vi "save_xml.vi"(8 "error in":errorcluster, 10 "base path":path, 11 "Camera Setup":T1={"Analog Gain (0-5)"=4, "Exposure Time"=0.01, "EM Gain (0-255)"=0, "Trigger Polarity"="ATP P", "External Trigger Mode"="ATP P", "Scan Speed"="EMD E", "External Trigger Source"="SSP H", "Scan Mode"="ESC B", "Super Pixel Binning\n(if enabled in Scan Mode)"="SMD N", "Camera Sub-array acquisition region\n(if enabled in scan mode)"={"Left"=0, "Top"=0, "Width"=0, "Height"=0}, "Use camera?"=FALSE, "# image buffers"=100, "shots per measurement"=100, "Force images to U16"=FALSE, "Low Light Sensitivity"="LLS 0", "cooling"="CSW F", "fan"="FAN F", "Frame Grabber acquisition region"={"Left"=0, "Top"=0, "Right"=0, "Bottom"=0}} {"Frame Grabber acquisition region"."Bottom" max=512 step=1; "Frame Grabber acquisition region"."Right" max=512 step=1; "Frame Grabber acquisition region"."Top" max=512 step=1; "Frame Grabber acquisition region"."Left" max=512 step=1; "shots per measurement" min=0 step=1; "# image buffers" min=0 step=1; "Camera Sub-array acquisition region\n(if enabled in scan mode)"."Height" min=16 max=512 step=16; "Camera Sub-array acquisition region\n(if enabled in scan mode)"."Width" min=16 max=512 step=16; "Camera Sub-array acquisition region\n(if enabled in scan mode)"."Top" max=496 step=16; "Camera Sub-array acquisition region\n(if enabled in scan mode)"."Left" max=496 step=16; "Analog Gain (0-5)" max=5 step=1}) -> (0 "error out":errorcluster)   [LabVIEW 2013, in "Hamamatsu_C9100-13.lvclass"]
uses:
  Hamamatsu_C9100-13.lvclass
  <vilib>/Utility/xml.llb/Write to XML File(string).vi
  camera_setup.ctl
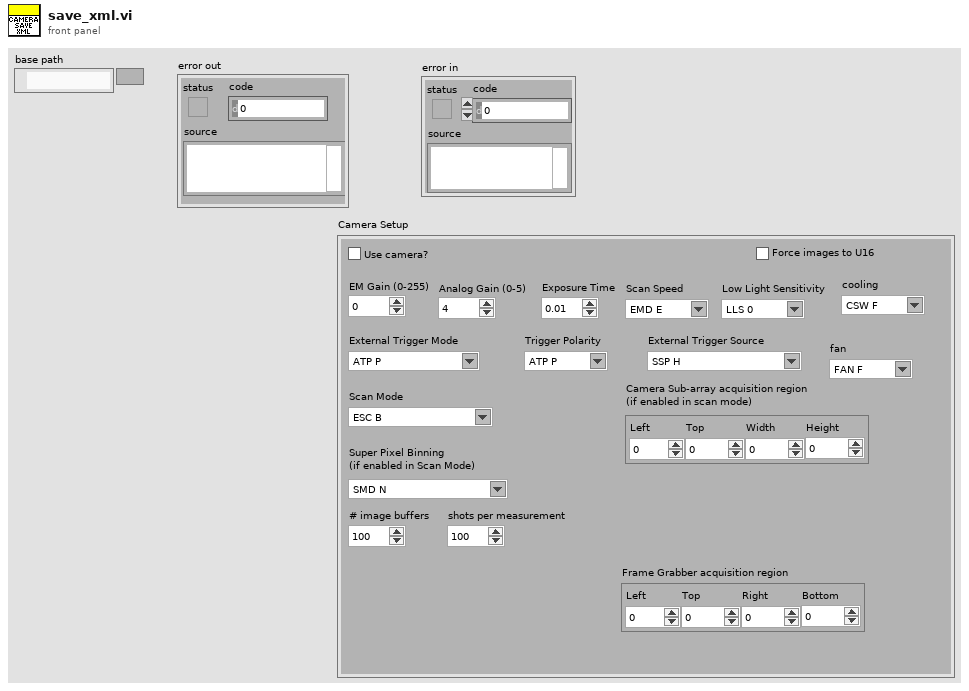
[diagram p1: front panel]
types:
  T1 = typedef "Hamamatsu_C9100-13.lvclass/camera_setup.ctl" = cluster{"Analog Gain (0-5)":u8, "Exposure Time":dbl, "EM Gain (0-255)":u8, "Trigger Polarity":string, "External Trigger Mode":string, "Scan Speed":string, "External Trigger Source":string, "Scan Mode":string, "Super Pixel Binning\n(if enabled in Scan Mode)":string, "Camera Sub-array acquisition region\n(if enabled in scan mode)":cluster{"Left":u16, "Top":u16, "Width":u16, "Height":u16}, "Use camera?":bool, "# image buffers":i32, "shots per measurement":i32, "Force images to U16":bool, "Low Light Sensitivity":string, "cooling":string, "fan":string, "Frame Grabber acquisition region":cluster{"Left":i32, "Top":i32, "Right":i32, "Bottom":i32}}
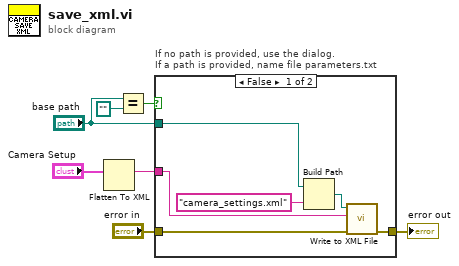
[diagram p0: block diagram]
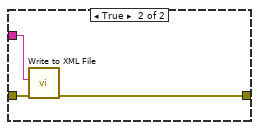
[diagram p2: hidden frame]
diagram:
  n1 = Flatten To XML(anything="Camera Setup") -> (xml string=w2:string)
  n2 = Equal?(x="base path", y=path "") -> (x = y?=w5:bool)
  n3 = case "If no path is provided, use the dialog.\nIf a path is provided, name file parameters.txt" shown="False" w5 {
    tunnel: [w9 w15] -> w6
    tunnel: "base path" -> [w12 _]
    tunnel: "error in" -> [w10 w16]
    tunnel: w2 -> [w8 w14]
    frame False {
      n4 = Build Path(base path=w12, name or relative path="camera_settings.xml") -> (appended path=w11:path)
      n5 = call-poly <vilib>:"Write to XML File.vi"("error in (no error)"=w10, "XML Input"=w8, "XML File Path"=w11) -> ("error out"=w9:errorcluster)  [unwired: 6 in, 2 out]
    }
    frame True {
      n6 = call-poly <vilib>:"Write to XML File.vi"("error in (no error)"=w16, "XML Input"=w14) -> ("error out"=w15:errorcluster)  [unwired: 7 in, 2 out]
    }
  }
  "error out" <- w6
